vi "Z Aux Direct Set Invert In.vi"(8 "error in (no error)":errorcluster caption="错误输入（无错误）", 9 "bifInvert":i32, 10 "ionum":i32, 11 "handle":u32) -> (0 "error out":errorcluster caption="错误输出", 2 "function return":i32, 3 "handle out":u32)   [LabVIEW 2019, in "zauxdll.lvlib"]
doc: "int32 __stdcall ZAux_Direct_SetInvertIn(ZMC_HANDLE handle, int ionum, int bifInvert);"
uses:
  zauxdll.lvlib
  zauxdll.dll
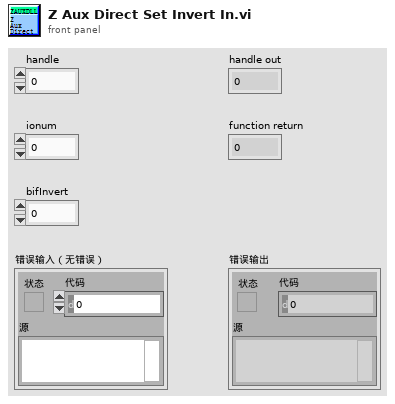
[diagram p1: front panel]
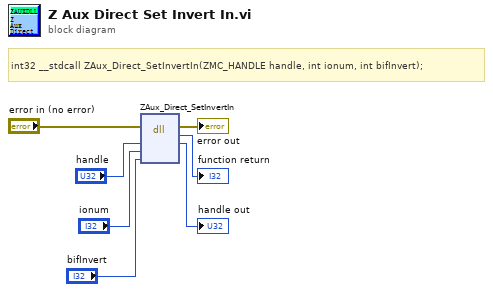
[diagram p0: block diagram]
diagram:
  # "int32 __stdcall ZAux_Direct_SetInvertIn(ZMC_HANDLE handle, int ionum, int bifInvert);"
  n1 = dll-call lib="C:/Users/VIC/Desktop/Standar Program/System/LLB/zmotion/zaux/zauxdll.*" fn="ZAux_Direct_SetInvertIn"(error in="error in (no error)", "handle"="handle", "ionum"="ionum", "bifInvert"="bifInvert") -> (error out=→"error out":errorcluster, →"function return":i32, "handle"=→"handle out":u32)  [unwired: 4 in, 1 out]
